vi "Autotuning PID (LabVIEW).vi"() -> ()   [LabVIEW 2010]
uses:
  <vilib>/addons/control/pid/NI_PID_autopid.lvlib
panel:
  out "Out of Correction Range":bool
  in  "Difference Threshold":dbl
  out "Out of Safety Range":bool
  in  "Safety Threshold":i32
  out "Motor Position on Activation":i32
  in  "Activate Output":bool
  out "Loop Counter":i32
  in  "Stop":bool
  out "dt out (s)":dbl format="%.3f"
  out "PID gains out":T1={"proportional gain (Kc)"=1.0, "integral time (Ti, min)"=0.01, "derivative time (Td, min)"=0.0} {"derivative time (Td, min)" format="%.3f"; "integral time (Ti, min)" format="%.3f"; "proportional gain (Kc)" format="%.3f"}
  out "tuning completed?":bool
  out "output":dbl format="%.2f"
  in  "autotuning parameters":T2={"controller type"=1, "relay cycles"=3, "relay amplitude"=1.0, "control specification"=2, "PV noise level"=0.1} {"PV noise level" format="%.2f"; "control specification" items=["normal", "fast", "slow"]; "relay amplitude" format="%.2f"; "controller type" items=["PID", "PI", "P"]}
  in  "output range":cluster{"output high":dbl, "output low":dbl}={"output high"=100.0, "output low"=-100.0} {"output low" format="%.2f"; "output high" format="%.2f"}
  in  "autotune? (F)":bool
  in  "reinitialize? (F)":bool
  in  "dt (s)":dbl=-1.0 format="%.3f"
  in  "PID gains":T1={"proportional gain (Kc)"=1.0, "integral time (Ti, min)"=0.01, "derivative time (Td, min)"=0.0} {"derivative time (Td, min)" format="%.3f"; "integral time (Ti, min)" format="%.3f"; "proportional gain (Kc)" format="%.3f"}
  in  "Wavenumber Setpoint":dbl format="%.4f"
  in  "Thick Etalon Position Setpoint":i32
  out "WS7 Ch1 Wavenumber":dbl format="%.4f"
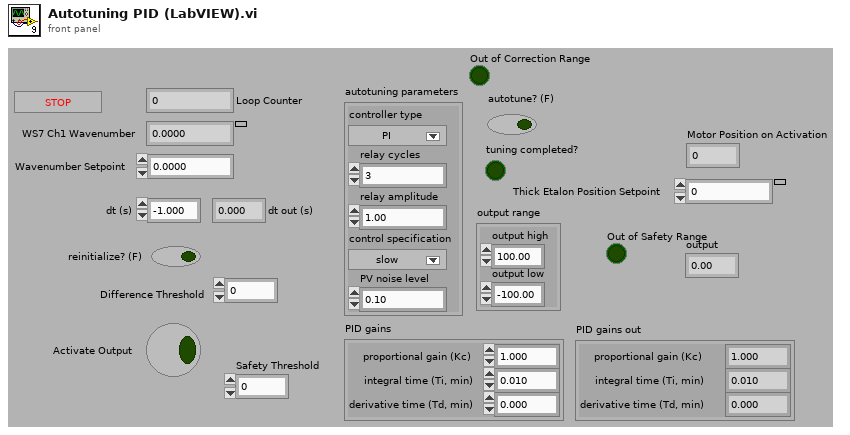
[diagram p1: front panel]
types:
  T1 = cluster{"proportional gain (Kc)":dbl, "integral time (Ti, min)":dbl, "derivative time (Td, min)":dbl}
  T2 = cluster{"controller type":u16, "relay cycles":i32, "relay amplitude":dbl, "control specification":u16, "PV noise level":dbl}
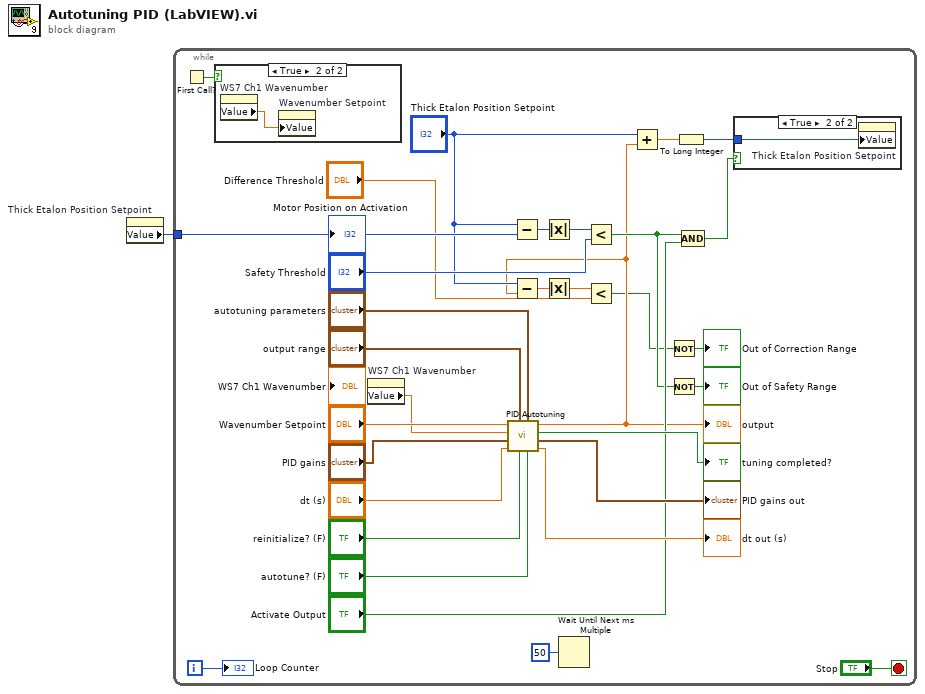
[diagram p0: block diagram]
diagram:
  n1 = property on="Thick Etalon Position Setpoint" class="DigNum (strict)"() -> ("Value"=w1:i32)  [unwired: 2 in, 2 out]
  n2 = while {
    tunnel: w1 -> [w16]
    i -> [w20]
    stop <- "Stop" stop-if-true
    n3 = First Call?() -> (First Call?: T/F=w33:bool)
    n4 = case shown="True" w33 {
      frame False {
      }
      frame True {
        n5 = property on="WS7 Ch1 Wavenumber" class="DigNum (strict)"() -> ("Value"=w35:dbl)  [unwired: 2 in, 2 out]
        n6 = property on="Wavenumber Setpoint" class="DigNum (strict)"("Value"=w35) -> ()  [unwired: 2 in, 2 out]
      }
    }
    n7 = property on="WS7 Ch1 Wavenumber" class="DigNum (strict)"() -> ("Value"=w31:dbl)  [unwired: 2 in, 2 out]
    n8 = call <vilib>:"PID Autotuning.vi"("autotune? (F)"="autotune? (F)", "autotuning parameters"="autotuning parameters", "reinitialize? (F)"="reinitialize? (F)", "output range"="output range", "dt (s)"="dt (s)", "PID gains"="PID gains", "process variable"=w31, "setpoint"="Wavenumber Setpoint") -> ("dt out (s)"=→"dt out (s)":dbl, "PID gains out"=→"PID gains out":T1, "tuning completed?"=→"tuning completed?":bool, "output"=w5:dbl)
    "output" <- w5
    n9 = Subtract(x="Thick Etalon Position Setpoint", y=w16) -> (x-y=w17:i32)
    n10 = Subtract(x="Thick Etalon Position Setpoint", y=w5) -> (x-y=w10:dbl)
    n11 = Absolute Value(x=w17) -> (abs(x)=w15:i32)
    n12 = Absolute Value(x=w10) -> (abs(x)=w11:dbl)
    n13 = Wait Until Next ms Multiple(millisecond multiple=u32 50) -> ()  [unwired: 1 out]
    n14 = Less?(x=w15, y="Safety Threshold") -> (x < y?=w13:bool)
    n15 = Less?(x=w11, y="Difference Threshold") -> (x < y?=w4:bool)
    n16 = Add(x="Thick Etalon Position Setpoint", y=w5) -> (x+y=w3:dbl)
    n17 = Not(x=w4) -> (.not. x?=→"Out of Correction Range":bool)
    n18 = Not(x=w13) -> (.not. x?=→"Out of Safety Range":bool)
    n19 = To Long Integer(number=w3) -> (32bit integer=w2:i32)
    n20 = Compound Arithmetic op=AND(w13, "Activate Output") -> (w12:bool)
    n21 = case shown="True" w12 {
      tunnel: w2 -> [_ w34]
      frame False {
      }
      frame True {
        n22 = property on="Thick Etalon Position Setpoint" class="DigNum (strict)"("Value"=w34) -> ()  [unwired: 2 in, 2 out]
      }
    }
    "Loop Counter" <- w20
    "Motor Position on Activation" <- w16
  }
